vi "oa_Create CIC LP Truncation Filter.vi"(9 "alias protect in final transition":bool, 11 "stop band attenuation":u16(ring)=2 items=["72 dB", "96 dB", "120 dB"]) -> (3 "lp filter settings":T1={"coefficients"=[], "factor"=1} {"coefficients" format="%.2f"})   [LabVIEW 2017, in "SoundVib_Resampling.lvlib"]
uses:
  <vilib>/addons/Sound and Vibration/Order Analysis/Resample Order Tracking/SoundVib_Resampling.lvlib
  <vilib>/addons/_NISVFA/_Shared subVIs/Controls/OAT Decimation Filter.ctl
  <vilib>/Analysis/2dsp.llb/Real FFT.vi
  <vilib>/Analysis/NI_AALPro.lvlib
panel:
  in  "Case Constant\n(See Context Help)":bool
  out "sum":dbl format="%_14e"
  in  "linear/log":bool
  out "frequency response":cluster{"Element Data":dbl, dbl, dbl[]}(graph)={"Element Data"=0.0, 1.52587890625e-05, []}
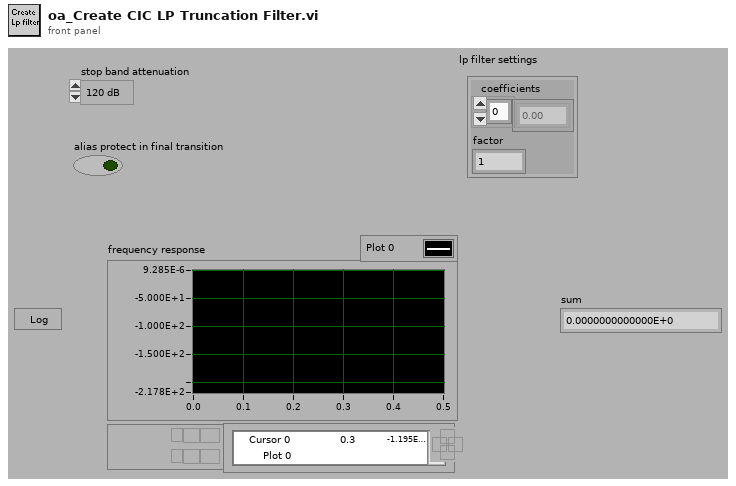
[diagram p1: front panel]
types:
  T1 = typedef "OAT Decimation Filter.ctl" = cluster{"coefficients":dbl[], "factor":i32}
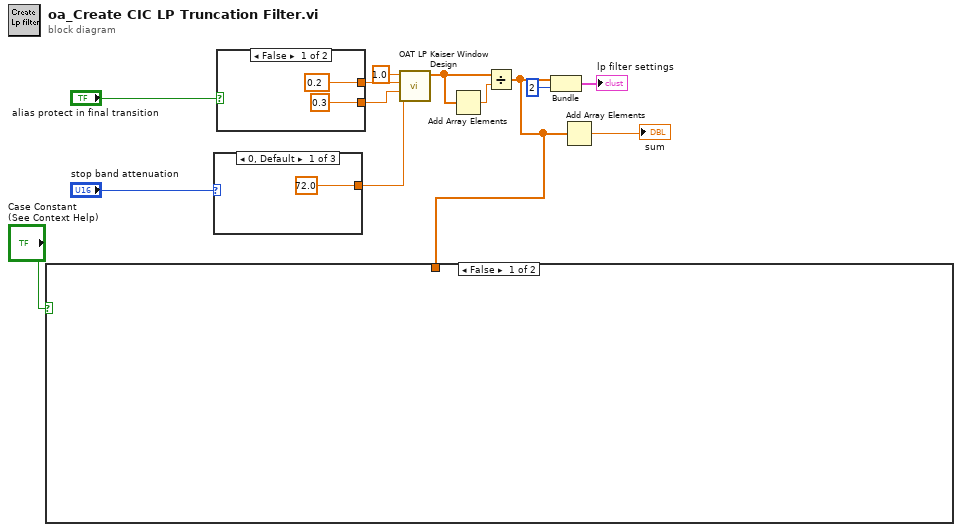
[diagram p0: block diagram]
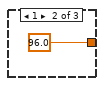
[diagram p2: hidden frame]
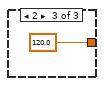
[diagram p3: hidden frame]
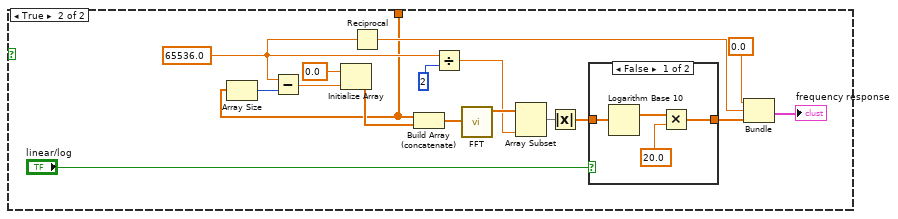
[diagram p4: hidden frame]
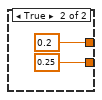
[diagram p6: hidden frame]
diagram:
  n1 = case shown="0, Default" "stop band attenuation" {
    tunnel: [72.0 ("Higher Freq") 96.0 ("Higher Freq") 120.0 ("Higher Freq")] -> w5
    frame 0, Default {
    }
    frame 1 {
    }
    frame 2 {
    }
  }
  n2 = case shown="False" "alias protect in final transition" {
    tunnel: [0.2 ("Higher Freq") 0.2 ("Higher Freq")] -> w8
    tunnel: [0.3 ("Higher Freq") 0.25 ("Higher Freq")] -> w7
    frame False {
    }
    frame True {
    }
  }
  n3 = call <vilib>:"OAT LP Kaiser Window Design.vi"("A stop [dB]"=w5, "stopband"=w7, "passband"=w8, "fs"=1.0) -> ("filter coefficients"=w2:dbl[])  [unwired: 5 in, 2 out]
  n4 = Add Array Elements(numeric array=w2) -> (sum=w4:dbl)
  n5 = Divide(x=w2, y=w4) -> (x/y=w1:dbl[])
  n6 = case shown="False" "Case Constant\n(See Context Help)" {
    tunnel: w1 -> [_ w21]
    frame False {
    }
    frame True {
      w22 = 65536.0 ("Element Data")
      n7 = Array Size(array=w21) -> (size(s)=w34:i32)
      n8 = Subtract(x=w22, y=w34) -> (x-y=w29:dbl)
      n9 = Initialize Array(0.0 ("Element Data"), w29) -> (w36:dbl[])
      n10 = Reciprocal(x=w22) -> (1/x=w25:dbl)
      n11 = Build Array (concatenate)(w21, w36) -> (w28:dbl[])
      n12 = Divide(x=w22, y=2) -> (x/y=w32:dbl)
      n13 = call-poly <vilib>:"FFT.vi"("X"=w28) -> ("FFT {X}"=w35:cdb[])  [unwired: 9 in, 1 out]
      n14 = Array Subset(array=w35, length=w32) -> (w31:cdb[])  [unwired: 1 in]
      n15 = Absolute Value(x=w31) -> (abs(x)=w23:dbl[])
      n16 = case shown="False" "linear/log" {
        tunnel: w23 -> [w41 w42]
        tunnel: [w40 w42] -> w26
        frame False {
          n17 = Logarithm Base 10(1:w41) -> (0:w39:dbl[])
          n18 = Multiply(x=w39, y=20.0 ("Element Data")) -> (x*y=w40:dbl[])
        }
        frame True {
        }
      }
      n19 = Bundle("Element Data"=0.0, w25, w26) -> (→"frequency response":cluster{"Element Data":dbl, dbl, dbl[]})  [unwired: 1 in]
    }
  }
  n20 = Bundle(w1, 2) -> (→"lp filter settings":cluster{dbl[], i32})  [unwired: 1 in]
  n21 = Add Array Elements(numeric array=w1) -> (sum=→"sum":dbl)
